vi "Convert mel to Hz.vi"(11 "mel":dbl) -> (3 "Hz":dbl)   [LabVIEW 2011]
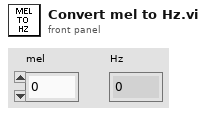
[diagram p1: front panel]
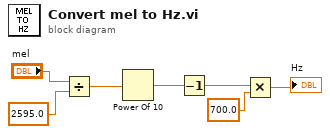
[diagram p0: block diagram]
diagram:
  n1 = Divide(x="mel", y=2595.0) -> (x/y=w3:dbl)
  n2 = Power Of 10(x=w3) -> (10^x=w4:dbl)
  n3 = Decrement(x=w4) -> (x-1=w5:dbl)
  n4 = Multiply(x=w5, y=700.0) -> (x*y=→"Hz":dbl)
